vi "Variant Attribute Lookup Table.vi"() -> ()   [LabVIEW 2023]
doc: "This example demonstrates building a variant attribute table that minimizes data copies when accessing the attribute values. Variant attribute tables are useful when you have a set of properties that you will lookup and modify by name."
uses:
  Lookup Table Data.ctl
panel:
  in  "Initial Value For New Attributes":T1=50
  in  "Stop":bool
  in  "Increment Amount":T1=10
  out "Attribute Value":T1
  in  "Increment":bool
  in  "Attribute Name":string
  # "Overview: This example demonstrates building a variant attribute table that minimizes data copies when accessing the attribute values. Variant attribute tables are useful when you have a set of properties that you will lookup and modify by name."
  # "Instructions"
  # "1. Choose a value for Initial Value For New Attributes before you run the VI.\n2. Run the VI.\n3. Type a name into Attribute Name. When you finish typing, the attribute value will be looked up. If it doesn't yet exist, it will be added with the specified Initial Value For New Attributes."
  # "4. Click Increment button to change the attribute's value.\n5. Repeat steps 2 and 3 for different attribute names, returning sometimes to previous attribute names. Each time you go back to an earlier name, the last value of that attribute will be retrieved from the lookup table.\n6. Press Stop to stop the VI.\n7. Review the block diagram for more details."
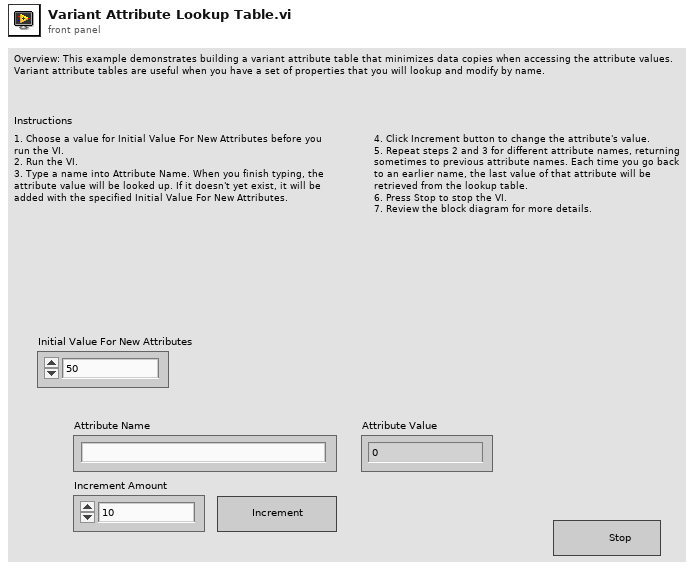
[diagram p1: front panel]
types:
  T1 = typedef "Lookup Table Data.ctl" = u32
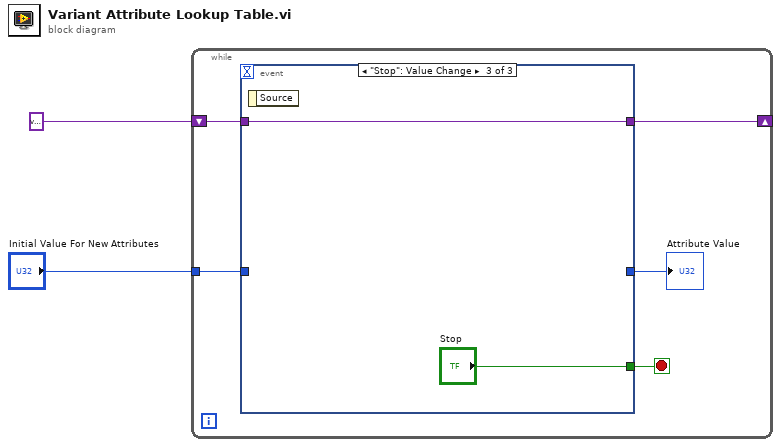
[diagram p0: block diagram]
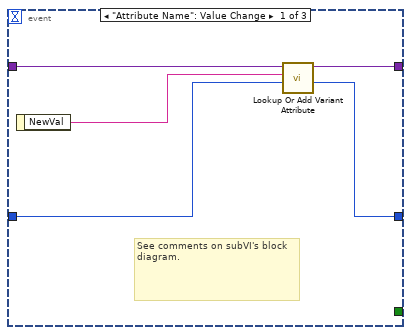
[diagram p2: hidden frame]
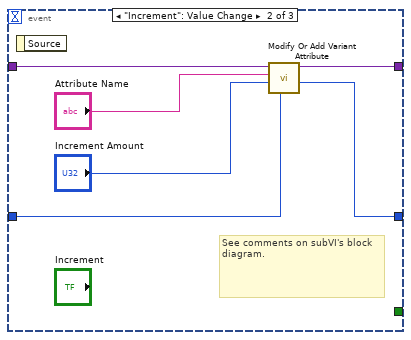
[diagram p3: hidden frame]
diagram:
  n1 = while {
    shift-right: [w6] -> _
    shift-left: variant -> [w7]
    tunnel: "Initial Value For New Attributes" -> [w3]
    stop <- w4 stop-if-true
    n2 = event shown="[2] \"Stop\": Value Change" {
      selector: _ -> [_ _ _]
      dyn-events: _ -> [_ _ _]
      timeout: _ -> [_ _ _]
      tunnel: w7 -> [w12 w18 w19]
      tunnel: [w11 w17 w19] -> w6
      tunnel: [w10 w15 _] -> w5
      tunnel: [_ _ "Stop"] -> w4
      tunnel: w3 -> [w8 w13 _]
      event "Attribute Name": Value Change {
        # "See comments on subVI's block diagram."
        n3 = event-data() -> ("NewVal"=w9:string)  [unwired: 1 in]
        n4 = call "Lookup Or Add Variant Attribute.vi"("Initial Value"=w8, "Attribute Name"=w9, "Variant in"=w12) -> ("Current Value"=w10:T1, "Variant out"=w11:variant)  [unwired: 6 in, 1 out]
      }
      event "Increment": Value Change {
        # "See comments on subVI's block diagram."
        n5 = event-data() -> ()  [unwired: 1 in, 1 out]
        n6 = call "Modify Or Add Variant Attribute.vi"("Initial Value For New Attributes"=w13, "Increment"="Increment Amount", "Attribute Name"="Attribute Name", "Variant in"=w18) -> ("Modified Attribute Value"=w15:T1, "Variant out"=w17:variant)  [unwired: 5 in, 1 out]
      }
      event "Stop": Value Change {
        n7 = event-data() -> ()  [unwired: 1 in, 1 out]
      }
    }
    "Attribute Value" <- w5
  }
